vi "Position error window.vi"(9 "Function":T1=enum."Window opened", 11 "Error Window ref":refnum<vi>) -> (0 "error out":errorcluster)   [LabVIEW 2020]
uses:
  Error window pos FGV states.ctl
  <vilib>/Utility/miscctls.llb/LVRectTypeDef.ctl
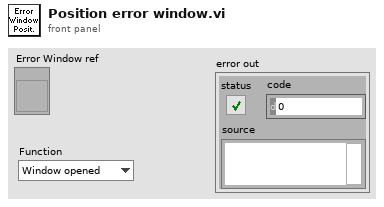
[diagram p1: front panel]
types:
  T1 = typedef "Error window pos FGV states.ctl" = enum16{"Read", "Window closed", "Window opened", "Reset"}
  T2 = typedef "LVRectTypeDef.ctl" = cluster{"Left":i16, "Top":i16, "Right":i16, "Bottom":i16}
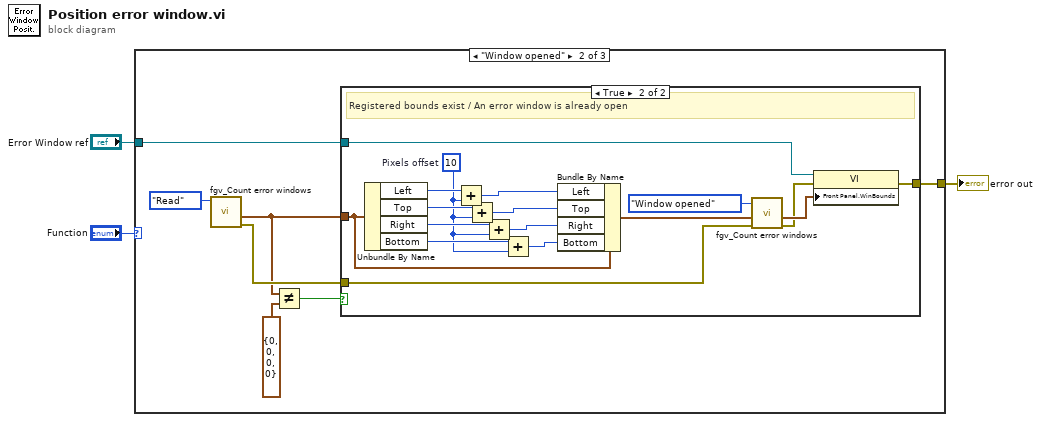
[diagram p0: block diagram]
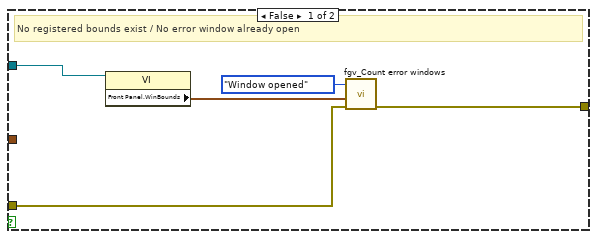
[diagram p3: hidden frame]
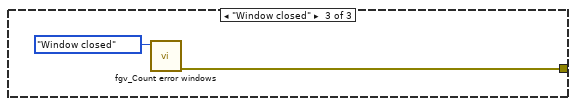
[diagram p4: hidden frame]
diagram:
  n1 = case shown="\"Window opened\"" "Function" {
    tunnel: "Error Window ref" -> [_ w9 _]
    tunnel: [_ w7 w33] -> w2
    frame Default {
    }
    frame "Window opened" {
      n2 = call "fgv_Count error windows.vi"("Function"=Error_window_pos_FGV_states."Read") -> ("error out"=w8:errorcluster, "Bounds of last error window"=w5:T2)  [unwired: 8 in, 1 out]
      n3 = Not Equal?(x=w5, y=T2 {"Left"=0, "Top"=0, "Right"=0, "Bottom"=0} ("Bounds of last error window")) -> (x != y?=w4:bool)
      n4 = case shown="True" w4 {
        tunnel: w9 -> [w12 w31]
        tunnel: w8 -> [w14 w20]
        tunnel: [w13 w19] -> w7
        tunnel: w5 -> [_ w16]
        frame False {
          # "No registered bounds exist / No error window already open"
          n5 = property on="Property Node" class="VI"(reference=w12) -> ("Front Panel.WinBounds"=w11:T2)  [unwired: 1 in, 2 out]
          n6 = call "fgv_Count error windows.vi"("error in (no error)"=w14, "Bounds of last error window"=w11, "Function"=Error_window_pos_FGV_states."Window opened") -> ("error out"=w13:errorcluster)  [unwired: 6 in, 2 out]
        }
        frame True {
          w22 = i16 10  # Pixels offset
          # "Registered bounds exist / An error window is already open"
          n7 = Unbundle By Name(w16) -> ("Left"=w30:i16, "Top"=w29:i16, "Right"=w28:i16, "Bottom"=w27:i16)
          n8 = Add(x=w30, y=w22) -> (x+y=w24:i16)
          n9 = Add(x=w29, y=w22) -> (x+y=w25:i16)
          n10 = Add(x=w28, y=w22) -> (x+y=w26:i16)
          n11 = Add(x=w27, y=w22) -> (x+y=w23:i16)
          n12 = Bundle By Name(cluster=w16, "Left"=w24, "Top"=w25, "Right"=w26, "Bottom"=w23) -> (w17:T2)
          n13 = call "fgv_Count error windows.vi"("error in (no error)"=w20, "Bounds of last error window"=w17, "Function"=Error_window_pos_FGV_states."Window opened") -> ("error out"=w18:errorcluster, "Bounds of last error window"=w21:T2)  [unwired: 6 in, 1 out]
          n14 = property on="Property Node" class="VI"(reference=w31, error in=w18, "Front Panel.WinBounds"=w21) -> (error out=w19:errorcluster)  [unwired: 1 out]
        }
      }
    }
    frame "Window closed" {
      n15 = call "fgv_Count error windows.vi"("Function"=Error_window_pos_FGV_states."Window closed") -> ("error out"=w33:errorcluster)  [unwired: 8 in, 2 out]
    }
  }
  "error out" <- w2
